vi "GEA3 Get Data ERD.vi"(8 "error in (no error)":errorcluster, 10 "Enable EMV List":bool, 11 ".NET Refnum in":refnum<k24>) -> (0 "error out":errorcluster, 1 "ERD Data":string[][](array[string]), 2 "ERD Data  2":T1, 3 ".NET Refnum out":refnum<k24>)   [LabVIEW 2016]
uses:
  C:/TechnologyLab/NI-2010/Drivers/GEA3 Toolkit/GEA3 DLL Source/GeaCommunication.dll
  GEA3 DLL Source/GeaCommunication.dll
  Type Definitions/GEA3 HEWH ERD Data.ctl
  Type Definitions/GEA3 HEWH Mixing Valve.ctl
  library/GEA2_Toolkit.lvlib
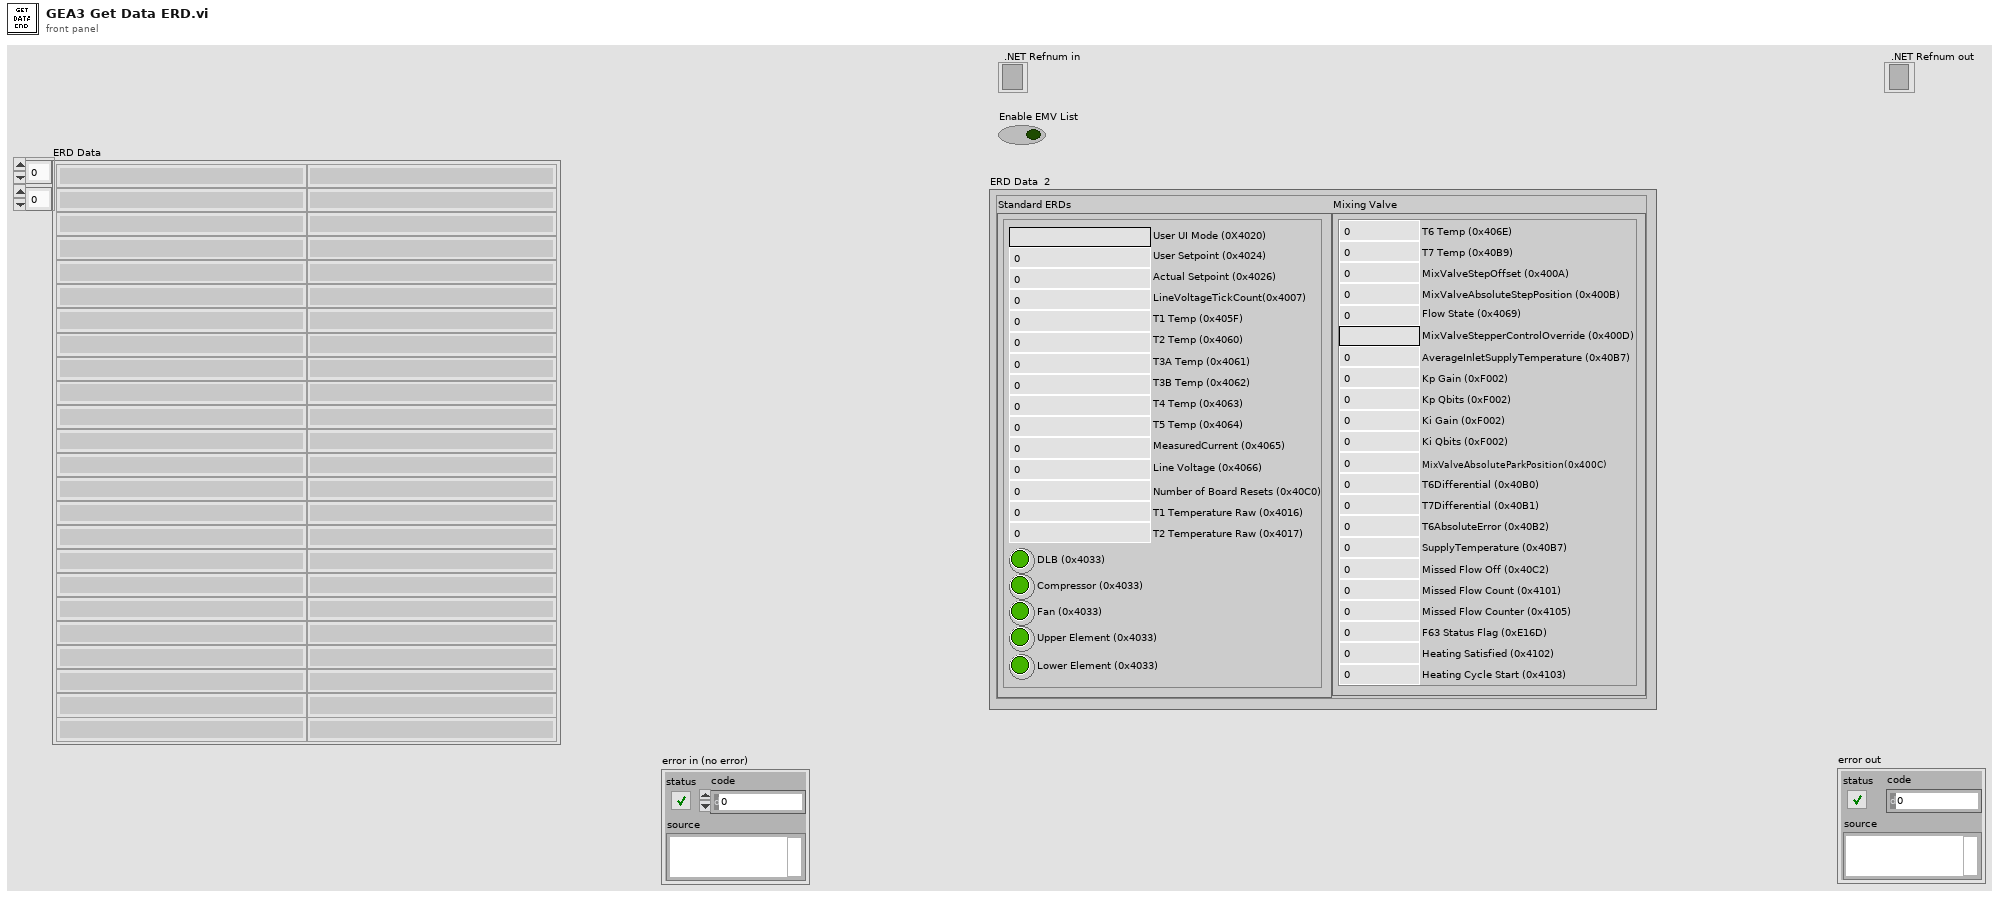
[diagram p1: front panel]
types:
  T1 = typedef "GEA3 HEWH ERD Data.ctl" = cluster{"Mixing Valve":T2, "Standard ERDs":cluster{"User UI Mode (0X4020)":string, "User Setpoint (0x4024)":u16, "Actual Setpoint (0x4026)":u16, "DLB (0x4033)":bool, "Compressor (0x4033)":bool, "Lower Element (0x4033)":bool, "Upper Element (0x4033)":bool, "Fan (0x4033)":bool, "T1 Temp (0x405F)":dbl, "T2 Temp (0x4060)":dbl, "T3A Temp (0x4061)":dbl, "T3B Temp (0x4062)":dbl, "T4 Temp (0x4063)":dbl, "T5 Temp (0x4064)":dbl, "Line Voltage (0x4066)":dbl, "MeasuredCurrent (0x4065)":dbl, "LineVoltageTickCount(0x4007)":u16, "Number of Board Resets (0x40C0)":u16, "T1 Temperature Raw (0x4016)":u16, "T2 Temperature Raw (0x4017)":u16}}
  T2 = typedef "GEA3 HEWH Mixing Valve.ctl" = cluster{"T7 Temp (0x40B9)":dbl, "MixValveStepOffset (0x400A)":i16, "MixValveAbsoluteStepPosition (0x400B)":i16, "Flow State (0x4069)":u8, "MixValveStepperControlOverride (0x400D)":string, "AverageInletSupplyTemperature (0x40B7)":dbl, "T6 Temp (0x406E)":dbl, "Kp Gain (0xF002)":u16, "Kp Qbits (0xF002)":u16, "Ki Gain (0xF002)":u16, "Ki Qbits (0xF002)":u16, "MixValveAbsoluteParkPosition(0x400C)":i16, "T7Differential (0x40B1)":dbl, "T6Differential (0x40B0)":dbl, "SupplyTemperature (0x40B7)":dbl, "Missed Flow Off (0x40C2)":u8, "T6AbsoluteError (0x40B2)":dbl, "Missed Flow Count (0x4101)":u16, "Missed Flow Counter (0x4105)":u16, "F63 Status Flag (0xE16D)":u16, "Heating Satisfied (0x4102)":u16, "Heating Cycle Start (0x4103)":u16}
  T3 = typedef "GEA2_Toolkit.lvlib/ERD Read Data In.ctl" = cluster{"ERD Number":u16, "Data Type":T4}
  T4 = typedef "GEA2_Toolkit.lvlib/Data Type.ctl" = enum16{"string", "boolean", "uint8_t", "uint16_t", "uint32_t", "uint64_t", "int8_t", "int16_t", "int32_t", "int64_t"}
  T5 = typedef "GEA2_Toolkit.lvlib/Source_Destination.ctl" = cluster{"Source":u8, "Destination":u8}
  T6 = typedef "GEA2_Toolkit.lvlib/ERD Read Data Out.ctl" = cluster{"ERD Number":u16, "Data":string}
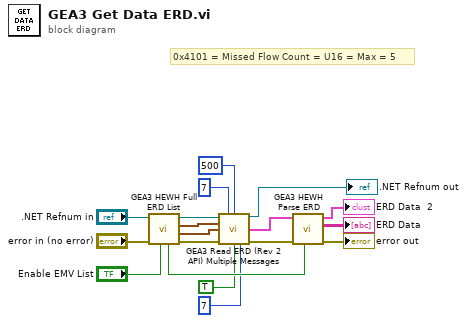
[diagram p0: block diagram]
diagram:
  # "0x4101 = Missed Flow Count = U16 = Max = 5"
  n1 = call "GEA3 HEWH Full ERD List.vi"("Enable EMV List"="Enable EMV List", "error in (no error)"="error in (no error)", "GEA2 Reference In"=".NET Refnum in") -> ("error out"=w12:errorcluster, "Read ERD List"=w14:T3[], "GEA Inputs"=w13:T5, "GEA2 Reference Out"=w16:refnum<k24>, "Enable EMV List"=w17:bool)  [unwired: 4 in]
  n2 = call "GEA3 Read ERD (Rev 2 API) Multiple Messages.vi"("GEA2 Reference In"=w16, "Retry Count"=7, "Read Timeout (ms)"=u32 500, "GEA Inputs"=w13, "Read ERD List"=w14, "Error In"=w12, "Verify ERD Response?"=TRUE, "Low Level Retry Count"=u8 7) -> ("GEA2 Reference Out"=→".NET Refnum out":refnum<k24>, "ERD Data Out"=w7:T6[], "Error Out"=w8:errorcluster)  [unwired: 4 in, 1 out]
  n3 = call "GEA3 HEWH Parse ERD.vi"("Enable EMV List?"=w17, "Error In"=w8, "ERD Data Out"=w7) -> ("Error Out"=→"error out":errorcluster, 2:"ERD Data"=→"ERD Data":string[][], 3:"ERD Data"=→"ERD Data  2":T1)  [unwired: 6 in]
